vi "Read Recipe List From File.vi"(8 "error in (no error)":errorcluster) -> (0 "error out":errorcluster, 3 "Recipe List":T1)   [LabVIEW 2021, in "Recipe.lvlib" / "Main Window.lvclass"]
uses:
  Main Window.lvclass
  Typedefs/Recipe List--cluster.ctl
  Recipe Window/Typedefs/Recipe Data--cluster.ctl
  Typedefs/Path--enum.ctl
  Main Window.lvclass/Main Window.ctl
  Recipe Window/Recipe Window.lvclass
  <vilib>/addons/_JKI.lib/Serialization/JSON/JKI JSON Serialization.lvlib
  <vilib>/Thomas ALLIBE/Path Utilities/Path Utilities.lvlib
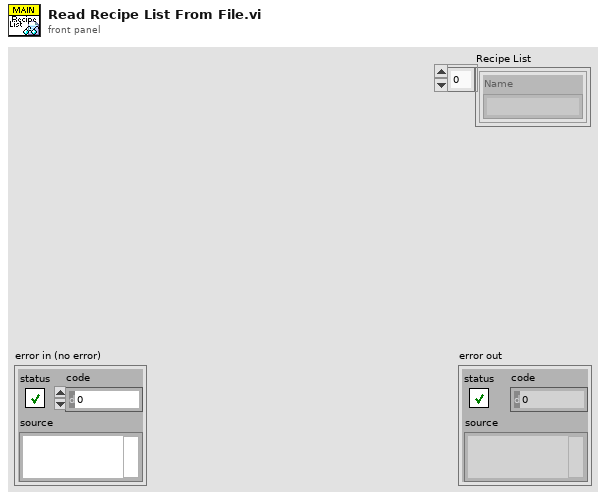
[diagram p1: front panel]
types:
  T1 = typedef "Recipe.lvlib/Main Window.lvclass/Recipe List--cluster.ctl" = T2[]
  T2 = typedef "Recipe.lvlib/Recipe Window.lvclass/Recipe Data--cluster.ctl" = cluster{"Name":string}
  T3 = typedef "Recipe.lvlib/Main Window.lvclass/Path--enum.ctl" = enum16{"Recipe List File"}
  T4 = enum16{"open", "replace", "create", "open or create", "replace or create", "replace or create with confirmation"}
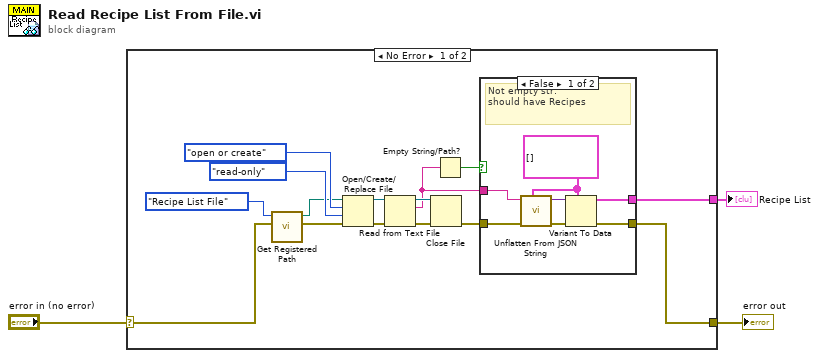
[diagram p0: block diagram]
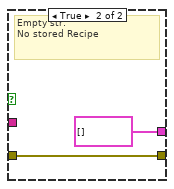
[diagram p2: hidden frame]
diagram:
  n1 = case shown="No Error" "error in (no error)" {
    selector: "error in (no error)" -> [w8 w28]
    tunnel: [w7 w28] -> w2
    tunnel: [w4 _] -> w1
    frame No Error {
      n2 = call <vilib>:"Get Registered Path.vi"("error in (no error)"=w8, "Key"=Path--enum."Recipe List File" ("Path")) -> ("error out"=w11:errorcluster, "Registered Path"=w10:path)  [unwired: 7 in, 1 out]
      n3 = Open/Create/Replace File(file path (use dialog)=w10, error in=w11, operation (0:open)=T4."open or create", access (0:read/write)=enum16{"read/write", "read-only", "write-only"}."read-only") -> (refnum out=w18:refnum<file>, error out=w17:errorcluster)  [unwired: 2 in, 1 out]
      n4 = Read from Text File(file (use dialog)=w18, error in=w17) -> (refnum out=w16:refnum<file>, text=w5:string, error out=w15:errorcluster)  [unwired: 2 in, 1 out]
      n5 = Close File(refnum=w16, error in=w15) -> (error out=w14:errorcluster)  [unwired: 1 out]
      n6 = Empty String/Path?(string/path=w5) -> (empty?=w6:bool)
      n7 = case shown="False" w6 {
        tunnel: w14 -> [w25 w26]
        tunnel: w5 -> [w24 _]
        tunnel: [w20 T1 [] ("Recipe List")] -> w4
        tunnel: [w19 w26] -> w7
        frame False {
          w21 = T1 [] ("Recipe List")
          # "Not empty str:\nshould have Recipes"
          n8 = call <vilib>:"Unflatten From JSON String.vi"("Type and Defaults"=w21, "error in (no error)"=w25, "JSON String"=w24) -> ("error out"=w23:errorcluster, "Variant"=w22:variant)  [unwired: 7 in]
          n9 = Variant To Data(error in=w23, type=w21, Variant=w22) -> (data=w20:T1, error out=w19:errorcluster)
        }
        frame True {
          # "Empty str:\nNo stored Recipe"
        }
      }
    }
    frame Error {
    }
  }
  "error out" <- w2
  "Recipe List" <- w1
